vi "APU Page - Multi FPGA.vi"(8 "error in (no error)":errorcluster, 11 "Node Ptr":T1 format="%.0x") -> (0 "error out":errorcluster)   [LabVIEW 2015, in "Engine Simulation Toolkit System Explorer.lvlib"]
uses:
  Engine Simulation Toolkit System Explorer.lvlib
  <vilib>/NI Veristand/Custom Device API/Custom Device Item Ref.ctl
  Shared/Properties.vi
  <vilib>/NI Veristand/Custom Device API/Get Item Property (U16).vi
  <vilib>/NI Veristand/Custom Device API/Get Item Property (Double).vi
  <vilib>/NI Veristand/Custom Device API/Get Item Property (String).vi
  <vilib>/NI Veristand/Custom Device API/Get Item Property (Boolean).vi
  Shared/Constants and GUIDs.vi
  <vilib>/NI Veristand/Custom Device Tools/Custom Device Utility Library/NI VeriStand - Search for Item by Name.vi
  <vilib>/NI Veristand/Custom Device API/Set Item Property (Double).vi
  <vilib>/NI Veristand/Custom Device API/Set Item Property (Boolean).vi
  <vilib>/NI Veristand/Custom Device API/Custom Device API.lvlib
  Shared/Engine Simulation Toolkit Shared.lvlib
  <vilib>/NI Veristand/Custom Device Tools/Custom Device Utility Library/Custom Device Utility Library.lvlib
panel:
  in  "Maximum angle deviation\nbetween RIO devices (degrees)":dbl
  out "RIO Devices":string
  in  "des speed":dbl caption="Start speed (RPM)"
  in  "Start angle (degrees)":dbl
  in  "des accel":dbl caption="Acceleration (RPM/sec)" min=0.0 format="%#_p"
  in  "Acceleration":bool
  out "Name in bitfile":string
  in  "Header":cluster{"Section Name":string}={"Section Name"="APU Settings"}
  in  "Description":string
  in  "Name":string
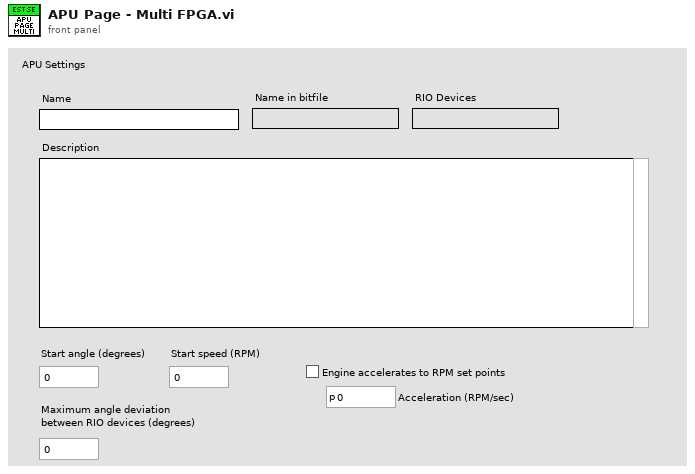
[diagram p1: front panel]
types:
  T1 = typedef "Custom Device API.lvlib/Custom Device Item Ref.ctl" = u64
  T2 = enum8{"Enabled", "Disabled", "Disabled and Grayed Out"}
  T3 = typedef "Engine Simulation Toolkit Shared.lvlib/Channel.ctl" = cluster{"Name":string, "Units":string, "Default":dbl, "Description":string, "Scalable":bool}
  T4 = typedef "Custom Device API.lvlib/Custom Device Channel.ctl" = cluster{"Type":T5, "Units":string, "Default Value":dbl, "Faultable":bool, "Scalable":bool}
  T5 = typedef "Custom Device API.lvlib/Custom Device Channel Type.ctl" = enum16{"Input", "Output"}
  T6 = typedef "Custom Device API.lvlib/Custom Device Item Info.ctl" = cluster{"Name":string, "Is Channel":bool, "GUID":string, "Is Waveform":bool}
  T7 = typedef "Custom Device API.lvlib/Custom Device Commands.ctl" = enum16{"Default", "Item renamed", "Shutdown", "Dynamic button pressed"}
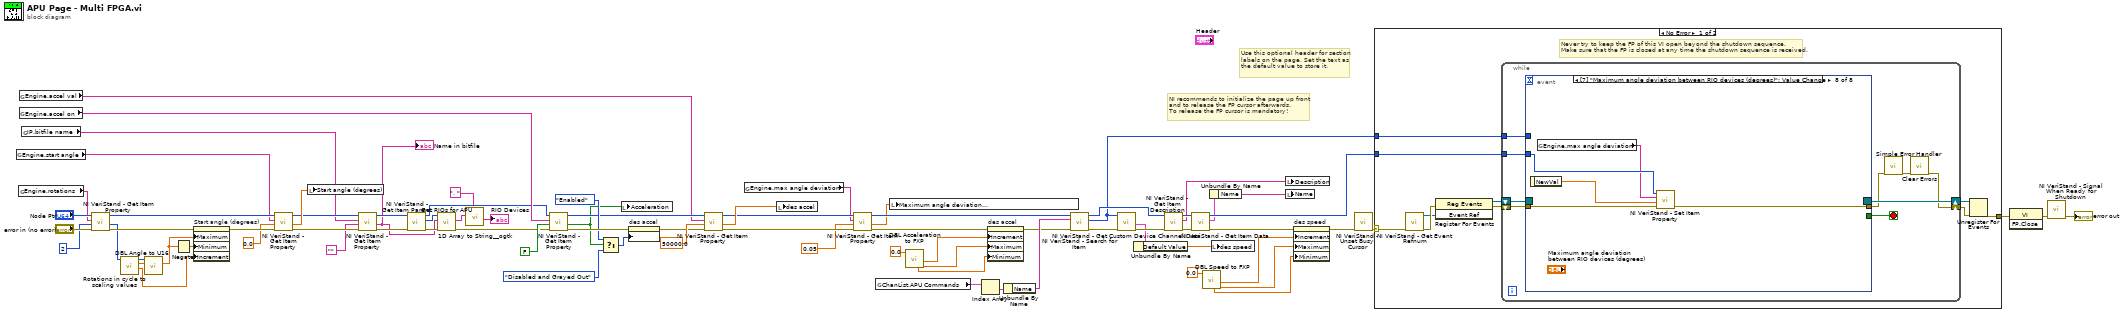
[diagram p0: block diagram]
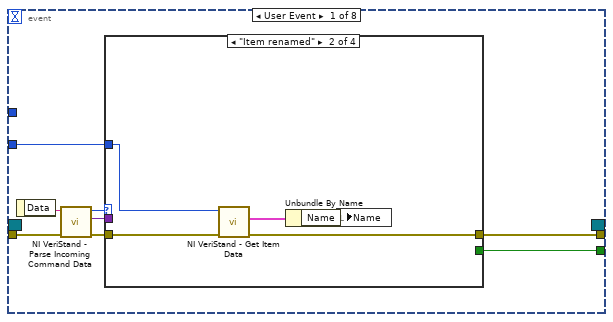
[diagram p2: hidden frame]
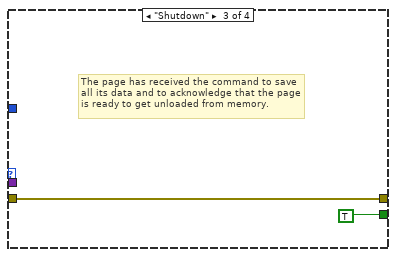
[diagram p4: hidden frame]
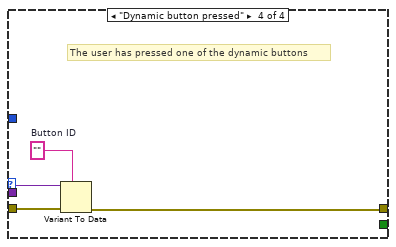
[diagram p5: hidden frame]
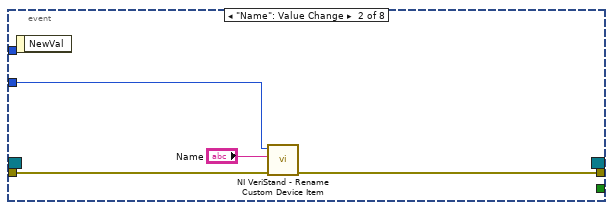
[diagram p6: hidden frame]
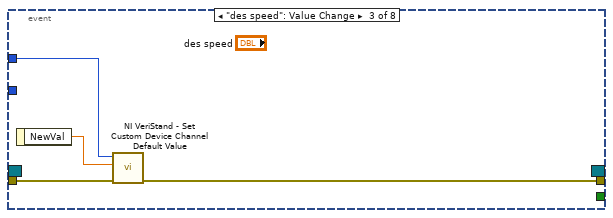
[diagram p7: hidden frame]
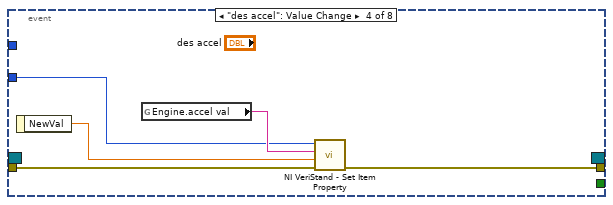
[diagram p8: hidden frame]
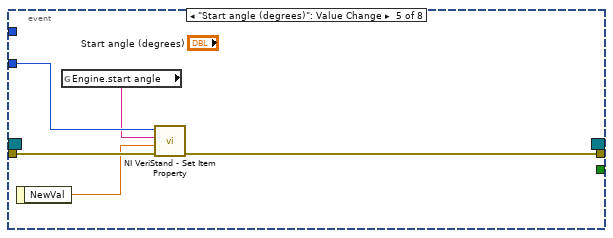
[diagram p9: hidden frame]
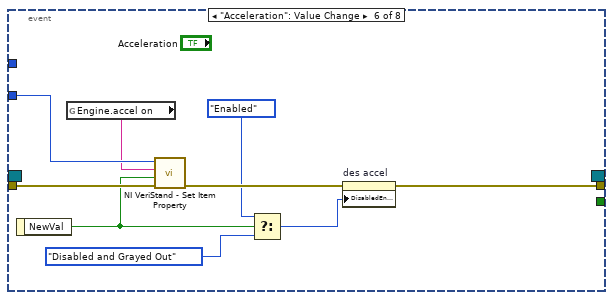
[diagram p10: hidden frame]
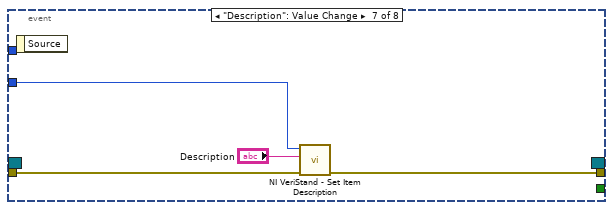
[diagram p11: hidden frame]
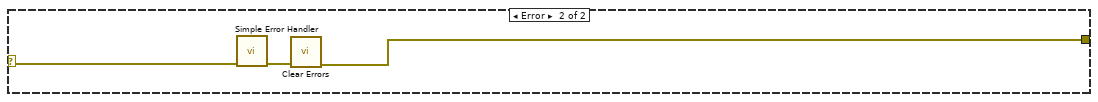
[diagram p12: hidden frame]
diagram:
  # "Use this optional header for section labels on the page. Set the text as the default value to store it."
  # "NI recommends to initialize the page up front\nand to release the FP cursor afterwards.\nTo release the FP cursor is mandatory!"
  n1 = global read "Properties.vi" "Engine.start angle"() -> (w62:string)
  n2 = global read "Properties.vi" "Engine.rotations"() -> (w66:string)
  n3 = global read "Properties.vi" "Engine.accel val"() -> (w49:string)
  n4 = global read "Properties.vi" "Engine.accel on"() -> (w55:string)
  n5 = global read "Properties.vi" "IP.bitfile name"() -> (w57:string)
  n6 = call-poly <vilib>:"NI VeriStand - Get Item Property.vi"("error in (no error)"="error in (no error)", "Default Value"=u16 2, "Property Name"=w66, "Item Ref in"="Node Ptr") -> ("error out"=w68:errorcluster, "Value"=w34:u16, "Item Ref out"=w63:T1)  [unwired: 4 in, 1 out]
  n7 = call "Rotations in cycle to scaling values.vi"("rotations in a cycle"=w34) -> ("degrees of one u16"=w30:dbl, "angle to u16 scale factor"=w32:dbl, "total angle span (degrees)"=w33:u16)  [unwired: 8 in]
  n8 = call "DBL Angle to U16.vi"("angle to u16 scale factor"=w32, "Desired angle (degrees)"=w33) -> ("Actual angle (degrees)"=w31:dbl)  [unwired: 8 in, 1 out]
  n9 = Negate(x=w31) -> (-x=w35:dbl)
  n10 = property on="Start angle (degrees)" class="DigNum (strict)"(error in=w68, "Maximum"=w31, "Minimum"=w35, "Increment"=w30) -> (error out=w61:errorcluster)  [unwired: 1 in, 1 out]
  n11 = call-poly <vilib>:"NI VeriStand - Get Item Property.vi"("error in (no error)"=w61, "Default Value"=0.0, "Property Name"=w62, "Item Ref in"=w63) -> ("error out"=w64:errorcluster, "Value"=w59:dbl, "Item Ref out"=w58:T1)  [unwired: 4 in, 1 out]
  n12 = local write "Start angle (degrees)"(w59) -> ()
  n13 = call-poly <vilib>:"NI VeriStand - Get Item Property.vi"("error in (no error)"=w64, "Default Value"="", "Property Name"=w57, "Item Ref in"=w58) -> ("error out"=w17:errorcluster, "Value"=w11:string, "Item Ref out"=w14:T1)  [unwired: 4 in, 1 out]
  "Name in bitfile" <- w11
  n14 = call <vilib>:"NI VeriStand - Get Item Parent.vi"("error in (no error)"=w17, "Item Ref in"=w14) -> ("error out"=w16:errorcluster, "Parent Ref"=w15:T1, "Item Ref out"=w13:T1)  [unwired: 6 in, 1 out]
  n15 = call "Get RIOs for APU.vi"("error in (no error)"=w16, "APU name"=w11, "Item Ref in"=w15) -> ("error out"=w12:errorcluster, "RIO Addresses"=w10:string[])  [unwired: 6 in, 1 out]
  n16 = call <userlib>:"1D Array to String__ogtk.vi"("delimiter (Tab)"=", ", "Array of Strings"=w10) -> ("delimited string"=→"RIO Devices":string)  [unwired: 9 in]
  n17 = call-poly <vilib>:"NI VeriStand - Get Item Property.vi"("error in (no error)"=w12, "Default Value"=FALSE, "Property Name"=w55, "Item Ref in"=w13) -> ("error out"=w53:errorcluster, "Value"=w36:bool, "Item Ref out"=w50:T1)  [unwired: 4 in, 1 out]
  n18 = Select(t=T2."Enabled" ("Disabled"), s=w36, f=T2."Disabled and Grayed Out" ("Disabled")) -> (s? t:f=w48:T2)
  n19 = local write "Acceleration"(w36) -> ()
  n20 = property on="des accel" class="DigNum (strict)"(error in=w53, "DisabledEnum"=w48) -> (error out=w18:errorcluster)  [unwired: 1 in, 1 out]
  n21 = call-poly <vilib>:"NI VeriStand - Get Item Property.vi"("error in (no error)"=w18, "Default Value"=50000.0, "Property Name"=w49, "Item Ref in"=w50) -> ("error out"=w7:errorcluster, "Value"=w46:dbl, "Item Ref out"=w6:T1)  [unwired: 4 in, 1 out]
  n22 = global read "Properties.vi" "Engine.max angle deviation"() -> (w2:string)
  n23 = local write "des accel"(w46) -> ()
  n24 = call-poly <vilib>:"NI VeriStand - Get Item Property.vi"("error in (no error)"=w7, "Default Value"=0.05, "Property Name"=w2, "Item Ref in"=w6) -> ("error out"=w5:errorcluster, "Value"=w3:dbl, "Item Ref out"=w4:T1)  [unwired: 4 in, 1 out]
  n25 = global read "Constants and GUIDs.vi" "ChanList.APU Commands"() -> (w44:T3[])
  n26 = local write "Maximum angle deviation\nbetween RIO devices (degrees)"(w3) -> ()
  n27 = call "DBL Acceleration to FXP.vi"("Desired acceleration (RPM/sec)"=0.0) -> ("accel max"=w22:dbl, "accel resolution"=w23:dbl, "accel min"=w21:dbl)  [unwired: 6 in, 2 out]
  n28 = Index Array(array=w44) -> (element=w43:T3)  [unwired: 1 in]
  n29 = property on="des accel" class="DigNum (strict)"(error in=w5, "Increment"=w23, "Maximum"=w22, "Minimum"=w21) -> (error out=w24:errorcluster)  [unwired: 1 in, 1 out]
  n30 = Unbundle By Name(w43) -> ("Name"=w42:string)
  n31 = call-poly <vilib>:"NI VeriStand - Search for Item.vi"("error in"=w24, "Item Name"=w42, "Section Ref in"=w4) -> ("error out"=w45:errorcluster, "Item Ref"=w37:T1, "Section Ref out"=w40:T1)  [unwired: 5 in, 1 out]
  n32 = call <vilib>:"NI VeriStand - Get Custom Device Channel Data.vi"("error in (no error)"=w45, "Channel Ref in"=w37) -> ("error out"=w41:errorcluster, "Channel"=w39:T4)  [unwired: 4 in, 4 out]
  n33 = Unbundle By Name(w39) -> ("Default Value"=w38:dbl)
  n34 = call <vilib>:"NI VeriStand - Get Item Description.vi"("error in (no error)"=w41, "Item Ref in"=w40) -> ("error out"=w71:errorcluster, "Description"=w72:string, "Item Ref out"=w73:T1)  [unwired: 7 out]
  n35 = call <vilib>:"NI VeriStand - Get Item Data.vi"("error in (no error)"=w71, "Item Ref in"=w73) -> ("error out"=w29:errorcluster, "Item Info"=w70:T6, "Item Ref out"=w74:T1)  [unwired: 7 out]
  n36 = call "DBL Speed to FXP.vi"("Desired speed (RPM)"=0.0) -> ("rpm max"=w26:dbl, "rpm resolution"=w27:dbl, "rpm min"=w25:dbl)  [unwired: 6 in, 2 out]
  n37 = Unbundle By Name(w70) -> ("Name"=w69:string)
  n38 = local write "des speed"(w38) -> ()
  n39 = local write "Description"(w72) -> ()
  n40 = local write "Name"(w69) -> ()
  n41 = property on="des speed" class="DigNum (strict)"(error in=w29, "Increment"=w27, "Maximum"=w26, "Minimum"=w25) -> (error out=w28:errorcluster)  [unwired: 1 in, 1 out]
  n42 = call <vilib>:"NI VeriStand - Unset Busy Cursor.vi"("error in (no error)"=w28) -> ("error out"=w76:errorcluster)  [unwired: 10 out]
  n43 = case shown="No Error" w76 {
    selector: w76 -> [w81 w157]
    tunnel: [w86 w155] -> w79
    tunnel: w74 -> [w82 _]
    tunnel: w37 -> [w80 _]
    frame No Error {
      # "Never try to keep the FP of this VI open beyond the shutdown sequence.\nMake sure that the FP is closed at any time the shutdown sequence is received."
      n44 = call <vilib>:"NI VeriStand - Get Event Refnum.vi"("error in (no error)"=w81) -> ("error out"=w89:errorcluster, "Event Ref"=w85:refnum<user-event>)  [unwired: 9 out]
      n45 = register-events(error in=w89, w85) -> (reference out=w83:refnum<event-registration>, error out=w84:errorcluster)  [unwired: 1 in]
      n46 = while {
        tunnel: w82 -> [w94]
        shift-right: [w91] -> w87
        shift-left: w84 -> [w97]
        shift-right: [w98] -> w88
        shift-left: w83 -> [w96]
        tunnel: w80 -> [w90]
        stop <- w95 stop-if-true
        n47 = event shown="[7] \"Maximum angle deviation between RIO devices (degrees)\": Value Change" {
          selector: w96 -> [_ _ _ _ _ _ _ _]
          dyn-events: [_ _ _ _ _ _ _ _] -> w98
          timeout: _ -> [_ _ _ _ _ _ _ _]
          tunnel: w97 -> [w106 w122 w126 w131 w136 w145 w148 w154]
          tunnel: [w102 _ _ _ _ _ _ _] -> w95
          tunnel: [w101 w121 w124 w130 w135 w137 w147 w153] -> w93
          tunnel: w94 -> [w100 w120 _ w127 w134 w144 w149 w152]
          tunnel: w90 -> [_ _ w125 _ _ _ _ _]
          event User Event {
            n48 = event-data() -> ("Data"=w105:string)  [unwired: 1 out]
            n49 = call <vilib>:"NI VeriStand - Parse Incoming Command Data.vi"("error in (no error)"=w106, "Incoming data"=w105) -> ("error out"=w104:errorcluster, "Outgoing data"=w99:variant, "Action"=w103:T7)  [unwired: 7 out]
            n50 = case shown="\"Item renamed\"" w103 {
              tunnel: w104 -> [w107 w112 w113 w118]
              tunnel: [_ _ TRUE _] -> w102
              tunnel: [w107 w109 w113 w115] -> w101
              tunnel: w100 -> [_ w111 _ _]
              tunnel: w99 -> [_ _ _ w117]
              frame "Default", Default {
              }
              frame "Item renamed" {
                n51 = call <vilib>:"NI VeriStand - Get Item Data.vi"("error in (no error)"=w112, "Item Ref in"=w111) -> ("error out"=w109:errorcluster, "Item Info"=w110:T6)  [unwired: 8 out]
                n52 = Unbundle By Name(w110) -> ("Name"=w108:string)
                n53 = local write "Name"(w108) -> ()
              }
              frame "Shutdown" {
                # "The page has received the command to save all its data and to acknowledge that the page is ready to get unloaded from memory."
              }
              frame "Dynamic button pressed" {
                w116 = ""  # Button ID
                # "The user has pressed one of the dynamic buttons"
                n54 = Variant To Data(error in=w118, type=w116, Variant=w117) -> (error out=w115:errorcluster)  [unwired: 1 out]
              }
            }
          }
          event "Name": Value Change {
            n55 = event-data() -> ()  [unwired: 2 out]
            n56 = call <vilib>:"NI VeriStand - Rename Custom Device Item.vi"("error in (no error)"=w122, "New Name"="Name", "Item Ref in"=w120) -> ("error out"=w121:errorcluster)  [unwired: 1 in, 7 out]
          }
          event "des speed": Value Change {
            n57 = event-data() -> ("NewVal"=w123:dbl)  [unwired: 1 out]
            n58 = call <vilib>:"NI VeriStand - Set Custom Device Channel Default Value.vi"("error in (no error)"=w126, "Default Value"=w123, "Channel Ref in"=w125) -> ("error out"=w124:errorcluster)  [unwired: 7 in, 1 out]
          }
          event "des accel": Value Change {
            n59 = event-data() -> ("NewVal"=w129:dbl)  [unwired: 1 out]
            n60 = global read "Properties.vi" "Engine.accel val"() -> (w128:string)
            n61 = call-poly <vilib>:"NI VeriStand - Set Item Property.vi"("error in (no error)"=w131, "Value"=w129, "Property Name"=w128, "Item Ref in"=w127) -> ("error out"=w130:errorcluster)  [unwired: 5 in, 2 out]
          }
          event "Start angle (degrees)": Value Change {
            n62 = event-data() -> ("NewVal"=w133:dbl)  [unwired: 1 out]
            n63 = global read "Properties.vi" "Engine.start angle"() -> (w132:string)
            n64 = call-poly <vilib>:"NI VeriStand - Set Item Property.vi"("error in (no error)"=w136, "Value"=w133, "Property Name"=w132, "Item Ref in"=w134) -> ("error out"=w135:errorcluster)  [unwired: 5 in, 2 out]
          }
          event "Acceleration": Value Change {
            n65 = event-data() -> ("NewVal"=w141:bool)  [unwired: 1 out]
            n66 = global read "Properties.vi" "Engine.accel on"() -> (w143:string)
            n67 = call-poly <vilib>:"NI VeriStand - Set Item Property.vi"("error in (no error)"=w145, "Value"=w141, "Property Name"=w143, "Item Ref in"=w144) -> ("error out"=w142:errorcluster)  [unwired: 5 in, 2 out]
            n68 = Select(t=T2."Enabled" ("Disabled"), s=w141, f=T2."Disabled and Grayed Out" ("Disabled")) -> (s? t:f=w139:T2)
            n69 = property on="des accel" class="DigNum (strict)"(error in=w142, "DisabledEnum"=w139) -> (error out=w137:errorcluster)  [unwired: 1 in, 1 out]
          }
          event "Description": Value Change {
            n70 = event-data() -> ()  [unwired: 2 out]
            n71 = call <vilib>:"NI VeriStand - Set Item Description.vi"("error in (no error)"=w148, "Description"="Description", "Item Ref in"=w149) -> ("error out"=w147:errorcluster)  [unwired: 8 out]
          }
          event "Maximum angle deviation\nbetween RIO devices (degrees)": Value Change {
            n72 = event-data() -> ("NewVal"=w151:dbl)  [unwired: 1 out]
            n73 = global read "Properties.vi" "Engine.max angle deviation"() -> (w150:string)
            n74 = call-poly <vilib>:"NI VeriStand - Set Item Property.vi"("error in (no error)"=w154, "Value"=w151, "Property Name"=w150, "Item Ref in"=w152) -> ("error out"=w153:errorcluster)  [unwired: 5 in, 2 out]
          }
        }
        n75 = call <vilib>:"Simple Error Handler.vi"("error in (no error)"=w93) -> ("error out"=w92:errorcluster)  [unwired: 1 in, 7 out]
        n76 = call <vilib>:"Clear Errors.vi"("error in (no error)"=w92) -> ("error out"=w91:errorcluster)  [unwired: 1 in, 5 out]
      }
      n77 = Unregister For Events(event registration refnum=w88, error in=w87) -> (error out=w86:errorcluster)
    }
    frame Error {
      n78 = call <vilib>:"Simple Error Handler.vi"("error in (no error)"=w157) -> ("error out"=w156:errorcluster)  [unwired: 1 in, 7 out]
      n79 = call <vilib>:"Clear Errors.vi"("error in (no error)"=w156) -> ("error out"=w155:errorcluster)  [unwired: 1 in, 5 out]
    }
  }
  n80 = invoke class="VI" method="FP.Close"(error in=w79) -> (error out=w78:errorcluster)  [unwired: 2 in, 2 out]
  n81 = call <vilib>:"NI VeriStand - Signal When Ready for Shutdown.vi"("error in (no error)"=w78) -> ("error out"=→"error out":errorcluster)  [unwired: 10 out]
